vi "Data_stream_read_test.vi"() -> ()   [LabVIEW 2018]
uses:
  <vilib>/Utility/miscctls.llb/LVPointTypeDef.ctl
  CTL_Test_state_contrlos.ctl
  <vilib>/Platform/TimedLoop/XDataNode/timing_clust.ctl
  <vilib>/Platform/TimedLoop/XDataNode/nitl_modes.ctl
  <vilib>/Platform/TimedLoop/XDataNode/wakeup.ctl
  <vilib>/Utility/error.llb/DialogType.ctl
  <vilib>/Utility/miscctls.llb/LVRGBAColorTypeDef.ctl
  <vilib>/Instr/_visa.llb/VISA Flush IO Buffer Mask.ctl
  <vilib>/Platform/TimedLoop/scheduler/LVUserAPI/_suppVIs/Create_1kHz_TSource.vi
  <vilib>/picture/3D Picture Control/Object/Create Object (name).vi
  <vilib>/picture/3D Picture Control/Object/Create Object (drawable).vi
  <vilib>/picture/3D Picture Control/Object/Add Object (reference).vi
  <vilib>/Instr/_visa.llb/VISA Configure Serial Port (Instr).vi
  <vilib>/platform/TimedLoop/XDataNode/XDataNode.xnode
  <vilib>/Platform/TimedLoop/XDataNode/XDNodeRunTimeDep.lvlib
  <vilib>/picture/3D Picture Control/NI_3D Picture Control.lvlib
panel:
  in  "Acq. data":bool
  in  "alpha":dbl(slide) scale=-180.0..180.0
  in  "Y":dbl(slide) scale=-90.0..90.0
  in  "X":dbl(slide) scale=-90.0..90.0
  out "Transform object refnum":refnum<vi>
  out "Mouse object refnum":refnum<vi>
  in  "Reset 3D view":bool
  in  "Target":cluster{"X":sgl, "Y":sgl, "Z":sgl}={"X"=0.0, "Y"=-0.01, "Z"=0.0} {"X" min=-10 max=10 step=0.01; "Y" min=-10 max=10 step=0.01; "Z" min=-10 max=10 step=0.01}
  in  "Camera Position":cluster{"X":sgl, "Y":sgl, "Z":sgl}={"X"=0.0, "Y"=-0.15, "Z"=0.2} {"X" min=-10 max=10 step=0.05; "Y" min=-10 max=10 step=0.05; "Z" min=-10 max=10 step=0.05}
  out "Cage object refnum":refnum<vi>
  in  "Automatic Projection Mode":enum16{"None", "Perspective", "Orthographic"}(ring)
  in  "Camera Controller:Type":T1(ring)=enum."Spherical"
  in  "3D Picture control":refnum<vi>(3d-picture)
  in  "error in (no error)":errorcluster
  in  "Serial port input":refnum<visa-resource-name>="COM6"
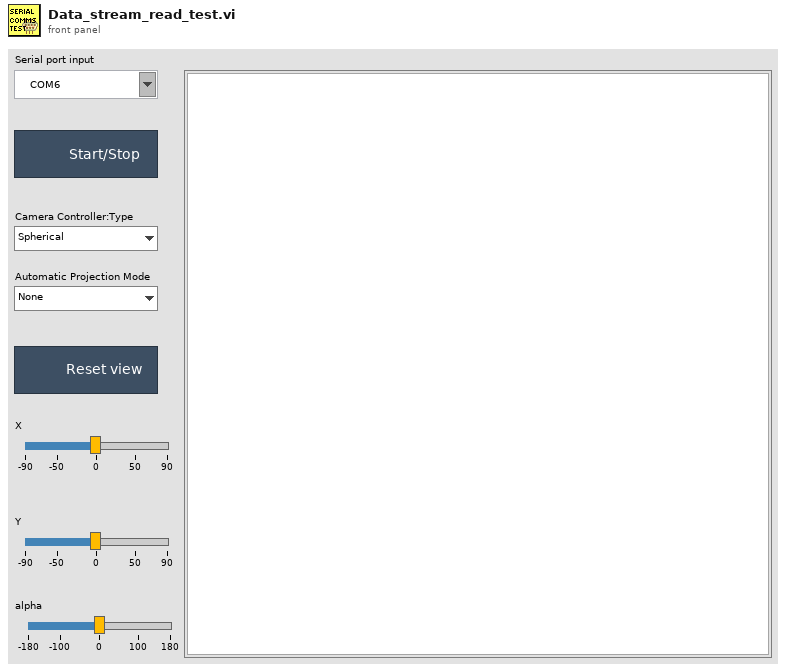
[diagram p1: front panel]
types:
  T1 = enum16{"None", "Spherical", "Flying", "Oriented"}
  T2 = typedef "LVPointTypeDef.ctl" = cluster{"Horizontal":i16, "Vertical":i16}
  T3 = typedef "CTL_Test_state_contrlos.ctl" = enum16{"Init", "Close App", "Play", "Stop", "3D params change", "Move mouse"}
  T4 = typedef "XDNodeRunTimeDep.lvlib/timing_clust.ctl" = cluster{"Expected End [f-1]":u64, "Actual End [f-1]":u64, "Finished Late? [f-1]":bool, "Expected End [i-1]":u64, "Actual End [i-1]":u64, "Finished Late? [i-1]":bool, "Expected Start [i]":u64, "Actual Start [i]":u64, "Expected Start [f]":u64, "Actual Start [f]":u64, "Source Name":string, "Structure Name":string, "Period":i64, "Deadline":i64, "Offset":i64, "Start":i64, "Priority":i32, "Timeout":i32, "Mode":T5, "Wakeup Reason":T6, "Error":errorcluster, "Source Type":string, "Secondary Source Type":string, "Global End Time":u64, "Global Start Time":u64, "Frame Duration":u64, "Iteration Duration":u64, "Assigned CPU":i32, "I/O Scan Engine Mode":u32}
  T5 = typedef "XDNodeRunTimeDep.lvlib/nitl_modes.ctl" = enum32{"No Change", "Process missed periods, maintain original phase", "Discard missed periods, maintain original phase", "Process missed periods, ignore original phase", "Discard missed periods, ignore original phase"}
  T6 = typedef "XDNodeRunTimeDep.lvlib/wakeup.ctl" = enum32{"Normal", "Aborted", "Asynchronous wakeup", "Timing source error", "Timed loop error", "Timeout"}
  T7 = enum16{"Inherit Material", "Use entire Material", "Ignore Ambient", "Ignore Diffuse", "Ignore Specular", "Ignore Emission", "Ignore Ambient and Diffuse"}
  T8 = typedef "LVRGBAColorTypeDef.ctl" = cluster{"Red":sgl, "Green":sgl, "Blue":sgl, "Alpha":sgl}
  T9 = typedef "DialogType.ctl" = u16
  T10 = enum32{"invalid app kind", "Development System", "Run Time System", "Student Edition", "Embedded LabVIEW", "Evaluation", "Custom"}
  T11 = typedef "VISA Flush IO Buffer Mask.ctl" = u16
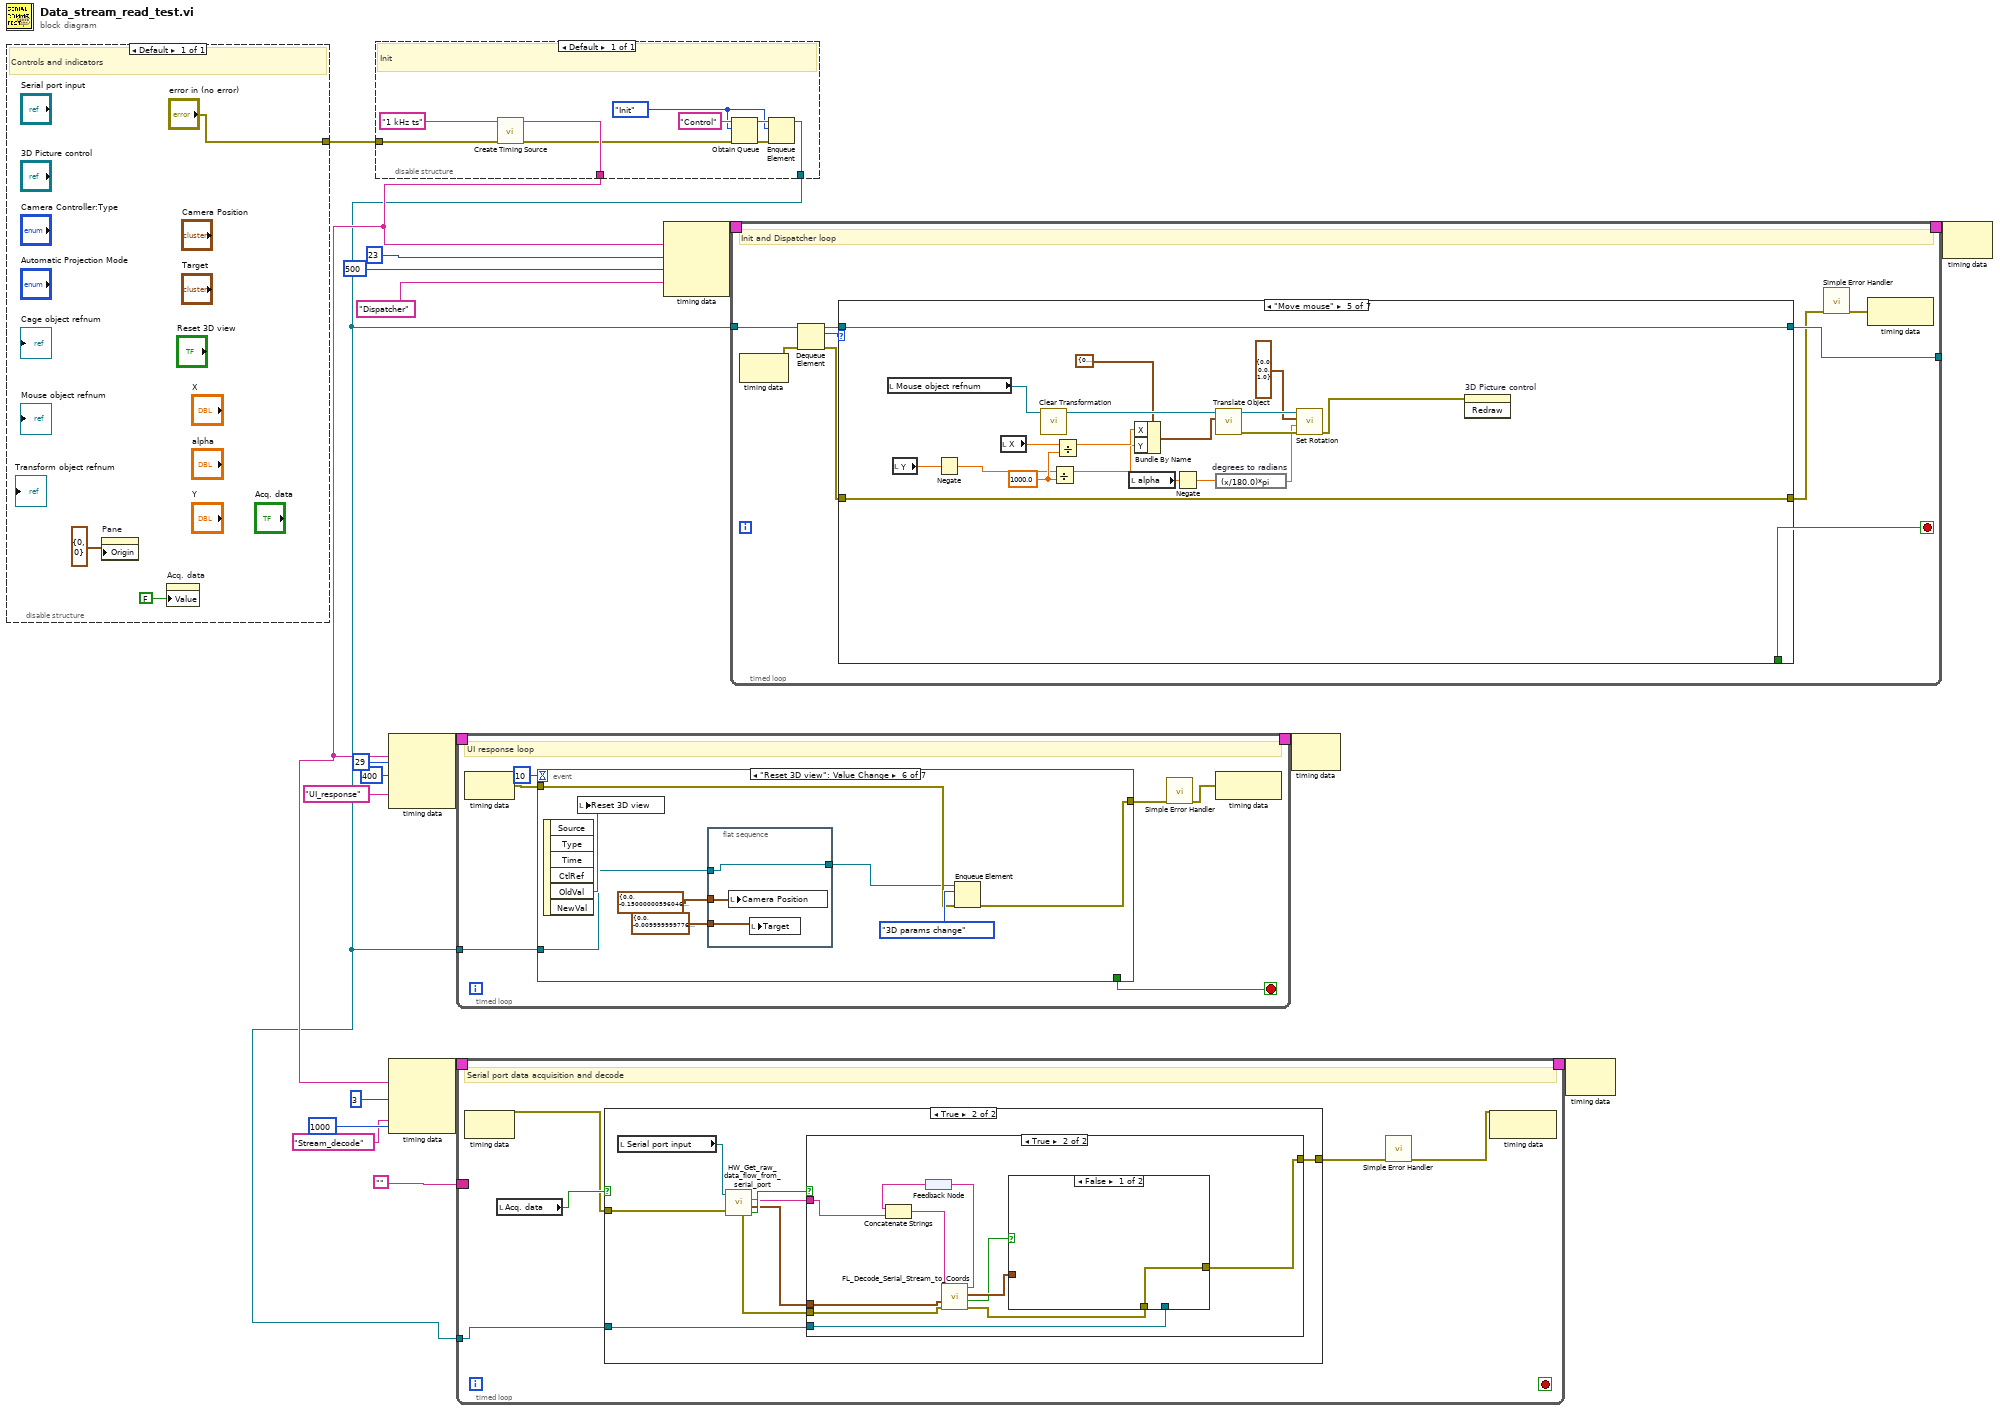
[diagram p0: block diagram]
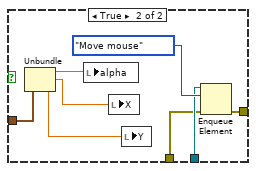
[diagram p4: hidden frame]
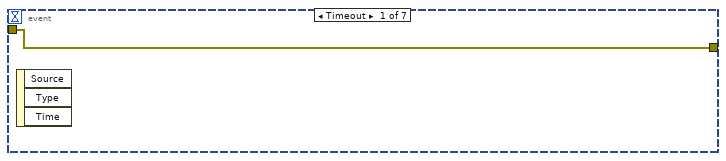
[diagram p5: hidden frame]
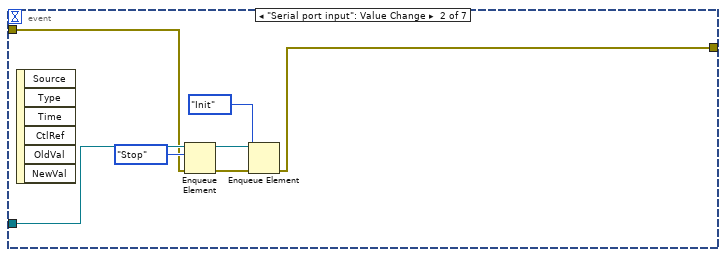
[diagram p6: hidden frame]
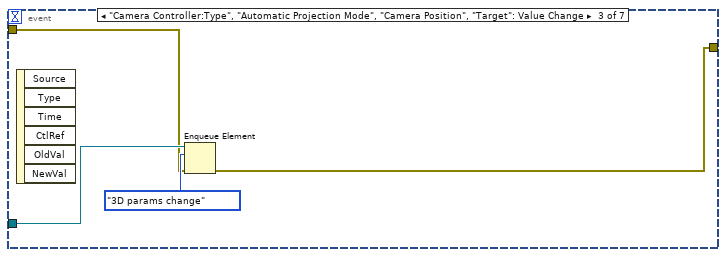
[diagram p7: hidden frame]
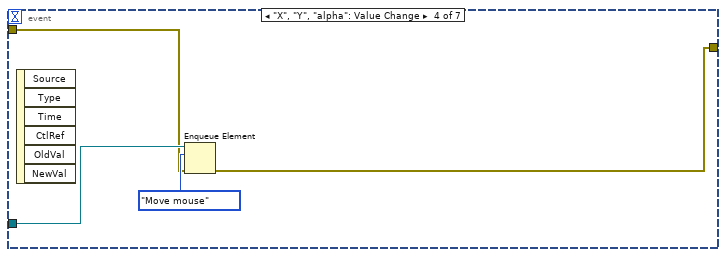
[diagram p8: hidden frame]
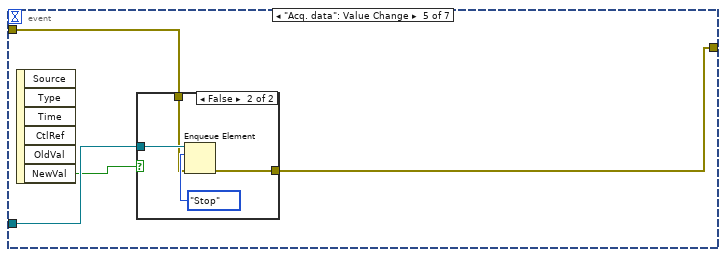
[diagram p9: hidden frame]
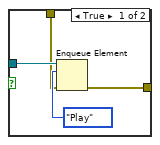
[diagram p10: hidden frame]
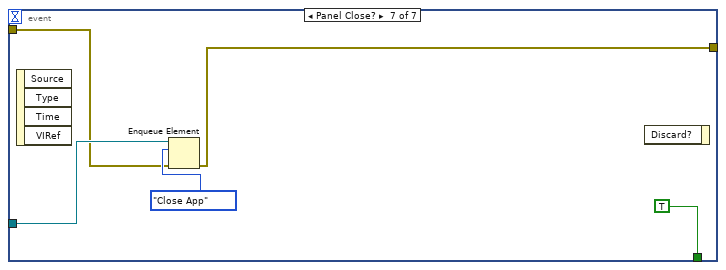
[diagram p11: hidden frame]
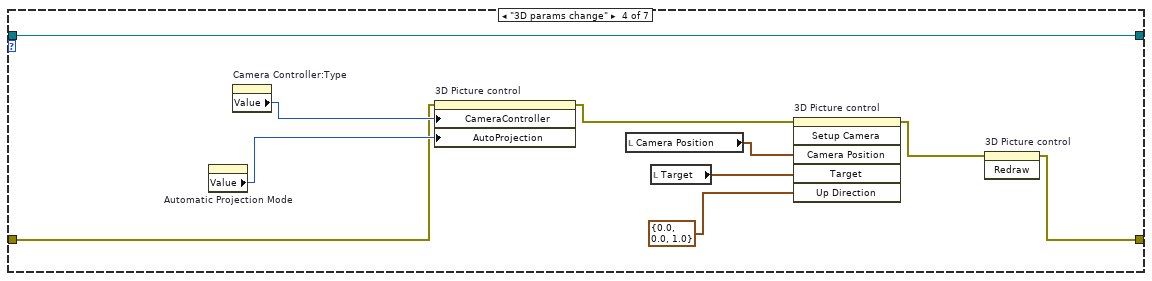
[diagram p15: hidden frame]
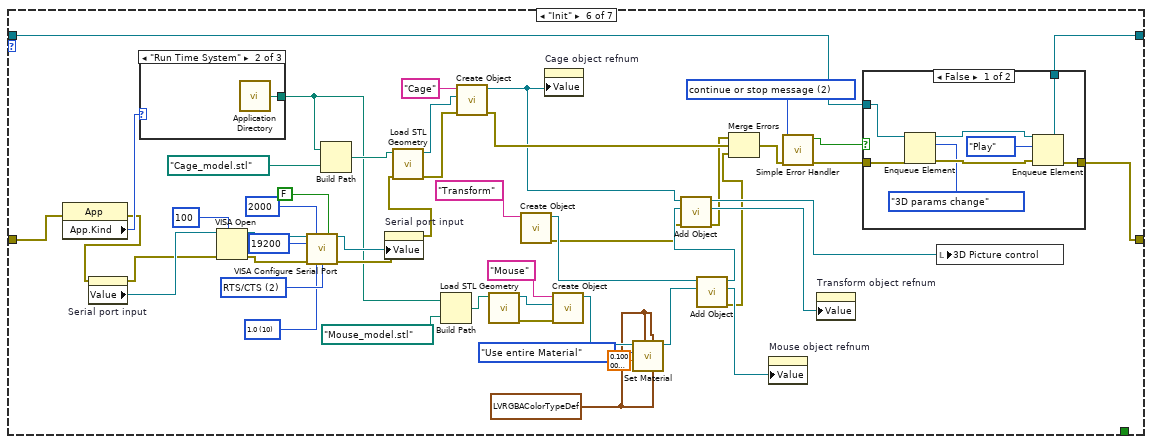
[diagram p16: hidden frame]
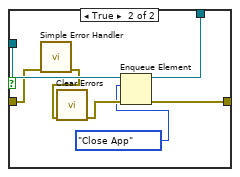
[diagram p17: hidden frame]
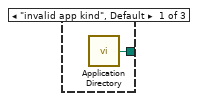
[diagram p18: hidden frame]
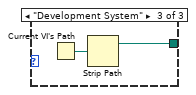
[diagram p19: hidden frame]
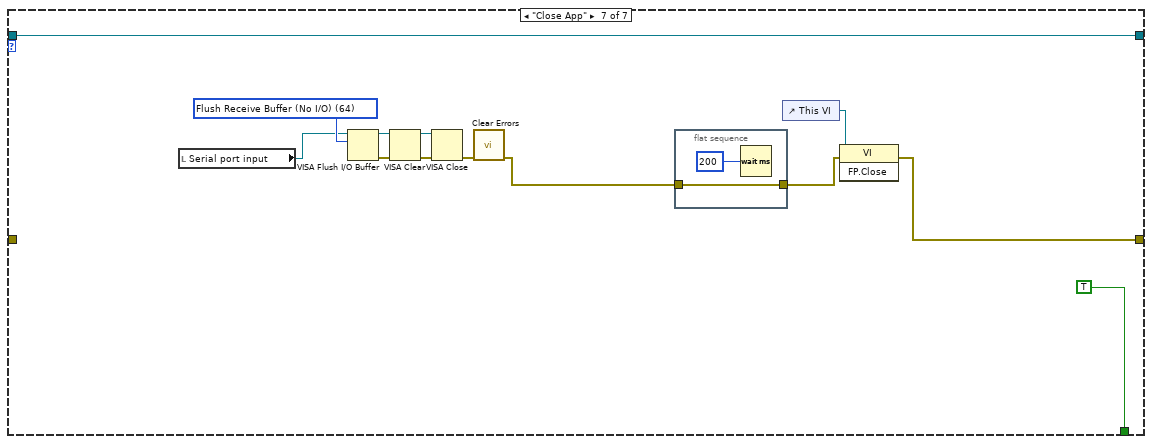
[diagram p20: hidden frame]
diagram:
  n1 = disable-structure shown="Default" {
    disable-tunnel: ["error in (no error)"] -> w19
    frame Enabled {
      # "Controls and indicators"
      n2 = property on="Pane" class="Pane"("Origin"=T2 {"Horizontal"=0, "Vertical"=0}) -> ()  [unwired: 2 in, 2 out]
      n3 = property on="Acq. data" class="Bool (strict)"("Value"=FALSE ("Acq. data")) -> ()  [unwired: 2 in, 2 out]
    }
  }
  n4 = disable-structure shown="Default" {
    disable-tunnel: w19 -> [w26]
    disable-tunnel: [w25] -> w1
    disable-tunnel: [w24] -> w6
    frame Enabled {
      w27 = CTL_Test_state_contrlos."Init"
      # "Init"
      n5 = call-poly <vilib>:"Create Timing Source.vi"("error in (no error)"=w26, "name (in)"="1 kHz ts") -> ("error out"=w23:errorcluster, "name (out)"=w24:string)  [unwired: 8 in]
      n6 = Obtain Queue(name (unnamed)="Control", element data type=w27, error in (no error)=w23) -> (queue out=w28:refnum<queue>, error out=w29:errorcluster)  [unwired: 2 in, 1 out]
      n7 = Enqueue Element(queue=w28, element=w27, error in (no error)=w29) -> (queue out=w25:refnum<queue>)  [unwired: 1 in, 2 out]
    }
  }
  n8 = node-c288(w6, i64 29 ("Period"), 400 ("Priority"), "UI_response" ("Structure Name")) -> (w13:T4)
  n9 = node-c288(w6, i64 3 ("Period"), 1000 ("Priority"), "Stream_decode" ("Structure Name")) -> (w8:T4)
  n10 = timed-loop {
    timing: w13 -> [_]
    timing-out: [_] -> w12
    tunnel: w1 -> [w36]
    stop <- w37 stop-if-true
    # "UI response loop"
    n11 = node-c288() -> (w33:errorcluster)  [unwired: 1 in]
    n12 = event shown="[5] \"Reset 3D view\": Value Change" {
      selector: _ -> [_ _ _ _ _ _ _]
      dyn-events: _ -> [_ _ _ _ _ _ _]
      timeout: 10 -> [_ _ _ _ _ _ _]
      tunnel: [_ _ _ _ _ _ TRUE] -> w37
      tunnel: w36 -> [_ w45 w49 w53 w57 w69 w80]
      tunnel: w33 -> [w38 w40 w47 w51 w56 w72 w78]
      tunnel: [w38 w39 w46 w50 w55 w71 w77] -> w32
      event Timeout {
        n13 = event-data() -> ()  [unwired: 1 in, 3 out]
      }
      event "Serial port input": Value Change {
        n14 = event-data() -> ()  [unwired: 1 in, 6 out]
        n15 = Enqueue Element(queue=w45, element=CTL_Test_state_contrlos."Stop", error in (no error)=w40) -> (queue out=w43:refnum<queue>, error out=w42:errorcluster)  [unwired: 1 in, 1 out]
        n16 = Enqueue Element(queue=w43, element=CTL_Test_state_contrlos."Init", error in (no error)=w42) -> (error out=w39:errorcluster)  [unwired: 1 in, 2 out]
      }
      event "Camera Controller:Type", "Automatic Projection Mode", "Camera Position", "Target": Value Change {
        n17 = event-data() -> ()  [unwired: 1 in, 6 out]
        n18 = Enqueue Element(queue=w49, element=CTL_Test_state_contrlos."3D params change", error in (no error)=w47) -> (error out=w46:errorcluster)  [unwired: 1 in, 2 out]
      }
      event "X", "Y", "alpha": Value Change {
        n19 = event-data() -> ()  [unwired: 1 in, 6 out]
        n20 = Enqueue Element(queue=w53, element=CTL_Test_state_contrlos."Move mouse", error in (no error)=w51) -> (error out=w50:errorcluster)  [unwired: 1 in, 2 out]
      }
      event "Acq. data": Value Change {
        n21 = event-data() -> ("NewVal"=w54:bool)  [unwired: 1 in, 5 out]
        n22 = case shown="False" w54 {
          tunnel: w57 -> [w61 w65]
          tunnel: w56 -> [w59 w63]
          tunnel: [w58 w62] -> w55
          frame True {
            n23 = Enqueue Element(queue=w61, element=CTL_Test_state_contrlos."Play", error in (no error)=w59) -> (error out=w58:errorcluster)  [unwired: 1 in, 2 out]
          }
          frame False {
            n24 = Enqueue Element(queue=w65, element=CTL_Test_state_contrlos."Stop", error in (no error)=w63) -> (error out=w62:errorcluster)  [unwired: 1 in, 2 out]
          }
        }
      }
      event "Reset 3D view": Value Change {
        n25 = event-data() -> ("OldVal"=w70:bool)  [unwired: 1 in, 5 out]
        n26 = local write "Reset 3D view"(w70) -> ()
        n27 = flat-sequence {
          tunnel: w69 -> [w76]
          tunnel: [w76] -> w68
          tunnel: cluster{"X":sgl, "Y":sgl, "Z":sgl} {"X"=0.0, "Y"=-0.15, "Z"=0.2} ("Camera Position") -> [w75]
          tunnel: cluster{"X":sgl, "Y":sgl, "Z":sgl} {"X"=0.0, "Y"=-0.01, "Z"=0.0} ("Target") -> [w74]
          frame #0 {
            n28 = local write "Camera Position"(w75) -> ()
            n29 = local write "Target"(w74) -> ()
          }
        }
        n30 = Enqueue Element(queue=w68, element=CTL_Test_state_contrlos."3D params change", error in (no error)=w72) -> (error out=w71:errorcluster)  [unwired: 1 in, 2 out]
      }
      event Panel Close? {
        n31 = event-data() -> ()  [unwired: 1 in, 4 out]
        n32 = Enqueue Element(queue=w80, element=CTL_Test_state_contrlos."Close App" ("State"), error in (no error)=w78) -> (error out=w77:errorcluster)  [unwired: 1 in, 2 out]
        n33 = event-data() -> ()  [unwired: 2 in, 1 out]
      }
    }
    n34 = call <vilib>:"Simple Error Handler.vi"("error in (no error)"=w32) -> ("error out"=w34:errorcluster)  [unwired: 4 in, 4 out]
    n35 = node-c288(w34) -> ()  [unwired: 1 out]
  }
  n36 = timed-loop {
    timing: w8 -> [_]
    timing-out: [_] -> w7
    border: "" ("Output string leftover") -> [_]
    tunnel: w1 -> [w89]
    stop <- _ stop-if-true
    # "Serial port data acquisition and decode"
    n37 = node-c288() -> (w90:errorcluster)  [unwired: 1 in]
    n38 = local read "Acq. data"() -> (w91:bool)
    n39 = case shown="True" w91 {
      tunnel: w90 -> [w92 w100]
      tunnel: w89 -> [_ w95]
      tunnel: [w92 w93] -> w88
      frame False {
      }
      frame True {
        n40 = local read "Serial port input"() -> (w97:refnum<visa-resource-name>)
        n41 = call "HW_Get_raw_data_flow_from_serial_port.vi"("error in"=w100, "VISA resource name in"=w97) -> ("Not empty?"=w99:bool, "error out"=w94:errorcluster, "Timestamp"=w96:timestamp, "Data"=w98:string)  [unwired: 2 in, 1 out]
        n42 = case shown="True" w99 {
          tunnel: w98 -> [_ w112]
          tunnel: w96 -> [_ w108]
          tunnel: w95 -> [_ w104]
          tunnel: w94 -> [w101 w107]
          tunnel: [w101 w102] -> w93
          frame False {
          }
          frame True {
            n43 = feedback #1() -> (w111:string)
            n44 = Concatenate Strings(w111, w112) -> (w110:string)
            n45 = call "FL_Decode_Serial_Stream_to_Coords.vi"("Error In"=w107, "Input timestamp"=w108, "Input string"=w110) -> ("Error Out"=w103:errorcluster, "Full frame?"=w105:bool, "Cluster of data"=w106:cluster{"alpha":dbl, "X":dbl, "Y":dbl}, "Input string leftover"=w109:string)  [unwired: 3 in]
            n46 = feedback-in #1(w109) -> ()
            n47 = case shown="False" w105 {
              tunnel: w106 -> [_ w121]
              tunnel: w104 -> [_ w116]
              tunnel: w103 -> [w113 w115]
              tunnel: [w113 w114] -> w102
              frame False {
              }
              frame True {
                n48 = Unbundle(w121) -> ("alpha"=w120:dbl, "X"=w119:dbl, "Y"=w118:dbl)
                n49 = local write "alpha"(w120) -> ()
                n50 = local write "X"(w119) -> ()
                n51 = local write "Y"(w118) -> ()
                n52 = Enqueue Element(queue=w116, element=CTL_Test_state_contrlos."Move mouse", error in (no error)=w115) -> (error out=w114:errorcluster)  [unwired: 1 in, 2 out]
              }
            }
          }
        }
      }
    }
    n53 = call <vilib>:"Simple Error Handler.vi"("error in (no error)"=w88) -> ("error out"=w87:errorcluster)  [unwired: 4 in, 4 out]
    n54 = node-c288(w87) -> ()  [unwired: 1 out]
  }
  n55 = node-c288(w6, i64 23 ("Period"), 500 ("Priority"), "Dispatcher" ("Structure Name")) -> (w18:T4)
  n56 = timed-loop {
    timing: w18 -> [_]
    timing-out: [_] -> w17
    tunnel: w1 -> [w135]
    tunnel: [w132] -> _
    stop <- w131 stop-if-true
    # "Init and Dispatcher loop"
    n57 = node-c288() -> (w130:errorcluster)  [unwired: 1 in]
    n58 = Dequeue Element(queue=w135, error in (no error)=w130) -> (queue out=w133:refnum<queue>, element=w134:T3, error out=w129:errorcluster)  [unwired: 1 in, 1 out]
    n59 = case shown="\"Move mouse\"" w134 {
      tunnel: [w137 w139 w141 w151 w170 w215 w252] -> w132
      tunnel: w133 -> [w137 w139 w141 w151 w170 w216 w252]
      tunnel: [_ _ _ _ _ _ TRUE] -> w131
      tunnel: [w136 w138 w140 w142 w169 w213 w244] -> w128
      tunnel: w129 -> [w136 w138 w140 w148 w169 w212 _]
      frame Default {
      }
      frame "Play" {
      }
      frame "Stop" {
      }
      frame "3D params change" {
        n60 = property on="Automatic Projection Mode" class="Enum (strict)"() -> ("Value"=w149:enum16{"None", "Perspective", "Orthographic"})  [unwired: 2 in, 2 out]
        n61 = property on="Camera Controller:Type" class="Enum (strict)"() -> ("Value"=w150:T1)  [unwired: 2 in, 2 out]
        n62 = property on="3D Picture control" class="SceneGraphDisp (strict)"(error in=w148, "CameraController"=w150, "AutoProjection"=w149) -> (error out=w147:errorcluster)  [unwired: 1 in, 1 out]
        n63 = local read "Camera Position"() -> (w146:cluster{"X":sgl, "Y":sgl, "Z":sgl})
        n64 = local read "Target"() -> (w145:cluster{"X":sgl, "Y":sgl, "Z":sgl})
        n65 = invoke on="3D Picture control" class="SceneGraphDisp (strict)" method="Setup Camera"(error in=w147, "Camera Position"=w146, "Target"=w145, "Up Direction"=cluster{"X":sgl, "Y":sgl, "Z":sgl} {"X"=0.0, "Y"=0.0, "Z"=1.0}) -> (error out=w143:errorcluster)  [unwired: 2 in, 5 out]
        n66 = invoke on="3D Picture control" class="SceneGraphDisp (strict)" method="Redraw"(error in=w143) -> (error out=w142:errorcluster)  [unwired: 2 in, 2 out]
      }
      frame "Move mouse" {
        w162 = 1000.0 ("y")
        n67 = local read "Mouse object refnum"() -> (w161:refnum<vi>)
        n68 = local read "Y"() -> (w154:dbl)
        n69 = Negate(x=w154) -> (-x=w152:dbl)
        n70 = local read "X"() -> (w165:dbl)
        n71 = call <vilib>:"Clear Transformation.vi"("Object Refnum In"=w161) -> ("Object Refnum Out"=w168:refnum<vi>)  [unwired: 9 in, 1 out]
        n72 = Divide(x=w152, y=w162) -> (x/y=w163:dbl)
        n73 = Divide(x=w165, y=w162) -> (x/y=w164:dbl)
        n74 = local read "alpha"() -> (w157:dbl)
        n75 = Bundle By Name(cluster=cluster{"X":sgl, "Y":sgl, "Z":sgl} {"X"=0.0, "Y"=0.0, "Z"=0.0} ("Translation"), "X"=w164, "Y"=w163) -> (w166:cluster{"X":sgl, "Y":sgl, "Z":sgl})
        n76 = Negate(x=w157) -> (-x=w153:dbl)
        n77 = call <vilib>:"Translate Object.vi"("Translation"=w166, "Scene.Object In"=w168) -> ("error out"=w158:errorcluster, "Scene.Object Out"=w160:refnum<vi>)  [unwired: 8 in]
        n78 = expression code="(x/180.0)*pi" "degrees to radians"(w153) -> (w156:dbl)
        n79 = call <vilib>:"Set Rotation.vi"("error in (no error)"=w158, "Angle"=w156, "Axis"=cluster{"X":sgl, "Y":sgl, "Z":sgl} {"X"=0.0, "Y"=0.0, "Z"=1.0}, "Scene Object"=w160) -> ("error out"=w155:errorcluster)  [unwired: 6 in, 1 out]
        n80 = invoke on="3D Picture control" class="SceneGraphDisp (strict)" method="Redraw"(error in=w155) -> ()  [unwired: 2 in, 3 out]
      }
      frame "Init" {
        w172 = T8 {"Red"=0.2, "Green"=0.2, "Blue"=0.3, "Alpha"=0.0} ("Diffuse")
        w200 = u16 10 items=["1.0"=10, "1.5"=15, "2.0"=20] ("stop bits (10: 1 bit)")
        w204 = u16 2 items=["None", "XON/XOFF", "RTS/CTS", "XON/XOFF & RTS/CTS", "DTR/DSR", "XON/XOFF & DTR/DSR"] ("flow control (0:none)")
        w218 = T9 2 items=["no dialog", "OK message", "continue or stop message", "OK message + warnings", "continue/stop + warnings"] ("type of dialog (OK msg:1)")
        n81 = property class="App"(error in=w212) -> (error out=w209:errorcluster, "App.Kind"=w220:T10)  [unwired: 1 in, 1 out]
        n82 = property on="Serial port input" class="VISAName"(error in=w209) -> (error out=w208:errorcluster, "Value"=w210:refnum<visa-resource-name>)  [unwired: 1 in, 1 out]
        n83 = case shown="\"Run Time System\"" w220 {
          tunnel: [w236 w237 w238] -> w190
          frame "invalid app kind", Default {
            n84 = call <vilib>:"Application Directory.vi"() -> ("Application Directory"=w236:path)
          }
          frame "Run Time System" {
            n85 = call <vilib>:"Application Directory.vi"() -> ("Application Directory"=w237:path)
          }
          frame "Development System" {
            n86 = Current VI's Path() -> (path=w239:path)
            n87 = Strip Path(path=w239) -> (stripped path=w238:path)  [unwired: 1 out]
          }
        }
        n88 = VISA Open(timeout (0)=u32 100 ("VISA Open timeout (0)"), error in (no error)=w208, VISA resource name=w210) -> (VISA resource name=w207:refnum<visa-resource-name>, error out=w206:errorcluster)  [unwired: 2 in]
        n89 = call-poly "VISA Configure Serial Port"("VISA resource name"=w207, "timeout (10sec)"=u32 2000, "Enable Termination\nChar (T)"=FALSE ("Enable Termination\nChar (T)"), "baud rate (9600)"=u32 19200, "error in (no error)"=w206, "stop bits (10: 1 bit)"=w200, "flow control (0:none)"=w204) -> ("VISA resource name out"=w199:refnum<visa-resource-name>, "error out"=w198:errorcluster)  [unwired: 7 in]
        n90 = Build Path(base path=w190, name or relative path=path "Cage_model.stl") -> (appended path=w211:path)
        n91 = property on="Serial port input" class="VISAName"(error in=w198, "Value"=w199) -> (error out=w197:errorcluster)  [unwired: 1 in, 1 out]
        n92 = call <vilib>:"Load STL Geometry.vi"("error in (no error)"=w197, "Model File"=w211) -> ("error out"=w195:errorcluster, "New Mesh Refnum"=w186:refnum<vi>)  [unwired: 8 in]
        n93 = Build Path(base path=w190, name or relative path=path "Mouse_model.stl") -> (appended path=w191:path)
        n94 = call-poly <vilib>:"Create Object.vi"("error in (no error)"=w195, "Geometry"=w186, "Name"="Cage") -> ("error out"=w187:errorcluster, "Scene:New Object"=w184:refnum<vi>)  [unwired: 7 in]
        n95 = call <vilib>:"Load STL Geometry.vi"("Model File"=w191) -> ("error out"=w192:errorcluster, "New Mesh Refnum"=w193:refnum<vi>)  [unwired: 9 in]
        n96 = call-poly <vilib>:"Create Object.vi"("Name"="Transform") -> ("error out"=w176:errorcluster, "Scene:New Object"=w181:refnum<vi>)  [unwired: 9 in]
        n97 = property on="Cage object refnum" class="LVObjRef (strict)"("Value"=w184) -> ()  [unwired: 2 in, 2 out]
        n98 = call-poly <vilib>:"Create Object.vi"("error in (no error)"=w192, "Geometry"=w193, "Name"="Mouse") -> ("Scene:New Object"=w175:refnum<vi>)  [unwired: 7 in, 1 out]
        n99 = call <vilib>:"Set Material.vi"("Diffuse"=w172, "Specular"=w172, "Ambient"=w172, "Shininess"=sgl 0.1, "Color Mode"=T7."Use entire Material", "Scene Object In"=w175) -> ("Scene Object Out"=w174:refnum<vi>)  [unwired: 4 in, 1 out]
        n100 = call-poly <vilib>:"Add Object.vi"("New Object In"=w174, "Scene Object In"=w181) -> ("error out"=w177:errorcluster, "New Object Out"=w179:refnum<vi>, "Scene Object Out"=w180:refnum<vi>)  [unwired: 7 in]
        n101 = call-poly <vilib>:"Add Object.vi"("error in (no error)"=w176, "New Object In"=w180, "Scene Object In"=w184) -> ("error out"=w178:errorcluster, "New Object Out"=w182:refnum<vi>, "Scene Object Out"=w183:refnum<vi>)  [unwired: 6 in]
        n102 = Merge Errors(w178, w187, w177) -> (w194:errorcluster)
        n103 = property on="Mouse object refnum" class="LVObjRef (strict)"("Value"=w179) -> ()  [unwired: 2 in, 2 out]
        n104 = call <vilib>:"Simple Error Handler.vi"("type of dialog (OK msg:1)"=w218, "error in (no error)"=w194) -> ("error?"=w217:bool, "error out"=w214:errorcluster)  [unwired: 3 in, 3 out]
        n105 = property on="Transform object refnum" class="LVObjRef (strict)"("Value"=w182) -> ()  [unwired: 2 in, 2 out]
        n106 = case shown="False" w217 {
          tunnel: w216 -> [w223 w235]
          tunnel: [w228 w234] -> w215
          tunnel: w214 -> [w225 w232]
          tunnel: [w227 w233] -> w213
          frame False {
            n107 = Enqueue Element(queue=w223, element=CTL_Test_state_contrlos."3D params change", error in (no error)=w225) -> (queue out=w222:refnum<queue>, error out=w224:errorcluster)  [unwired: 1 in, 1 out]
            n108 = Enqueue Element(queue=w222, element=CTL_Test_state_contrlos."Play", error in (no error)=w224) -> (queue out=w228:refnum<queue>, error out=w227:errorcluster)  [unwired: 1 in, 1 out]
          }
          frame True {
            n109 = call <vilib>:"Simple Error Handler.vi"("error in (no error)"=w232) -> ("error out"=w231:errorcluster)  [unwired: 4 in, 4 out]
            n110 = call <vilib>:"Clear Errors.vi"("error in (no error)"=w231) -> ("error out"=w230:errorcluster)  [unwired: 5 in, 1 out]
            n111 = Enqueue Element(queue=w235, element=CTL_Test_state_contrlos."Close App" ("State"), error in (no error)=w230) -> (queue out=w234:refnum<queue>, error out=w233:errorcluster)  [unwired: 1 in, 1 out]
          }
        }
        n112 = local write "3D Picture control"(w183) -> ()
      }
      frame "Close App" {
        w246 = T11 64 items=["Flush Receive Buffer"=16, "Write Transmit Buffer to Device"=32, "Flush Receive Buffer (No I/O)"=64, "Flush Transmit Buffer"=128] ("Mask")
        n113 = local read "Serial port input"() -> (w240:refnum<visa-resource-name>)
        n114 = VISA Flush I/O Buffer(VISA resource name=w240, mask (16)=w246) -> (VISA resource name out=w247:refnum<visa-resource-name>, error out=w248:errorcluster)  [unwired: 1 in]
        n115 = VISA Clear(VISA resource name=w247, error in (no error)=w248) -> (VISA resource name out=w250:refnum<visa-resource-name>, error out=w249:errorcluster)
        n116 = VISA Close(VISA resource name=w250, error in (no error)=w249) -> (error out=w251:errorcluster)
        n117 = call <vilib>:"Clear Errors.vi"("error in (no error)"=w251) -> ("error out"=w242:errorcluster)  [unwired: 5 in, 1 out]
        n118 = flat-sequence {
          tunnel: w242 -> [w253]
          tunnel: [w253] -> w243
          frame #0 {
            n119 = Wait (ms)(milliseconds to wait=u32 200) -> ()  [unwired: 1 out]
          }
        }
        n120 = control-ref of="This VI"() -> (w241:refnum<vi>)
        n121 = invoke class="VI" method="FP.Close"(reference=w241, error in=w243) -> (error out=w244:errorcluster)  [unwired: 1 in, 2 out]
      }
    }
    n122 = call <vilib>:"Simple Error Handler.vi"("error in (no error)"=w128) -> ("error out"=w127:errorcluster)  [unwired: 4 in, 4 out]
    n123 = node-c288(w127) -> ()  [unwired: 1 out]
  }
  n124 = node-c288(w12) -> ()  [unwired: 1 out]
  n125 = node-c288(w7) -> ()  [unwired: 1 out]
  n126 = node-c288(w17) -> ()  [unwired: 1 out]
